vi "synchronize with binary serial stream.vi"() -> ()   [LabVIEW 2017]
uses:
  typedefs/reading.ctl
  typedefs/readingType.ctl
  typedefs/bytes in a reading.ctl
panel:
  out "first reading":T1
  in  "error in":errorcluster
  in  "serial port":refnum<visa-resource-name>
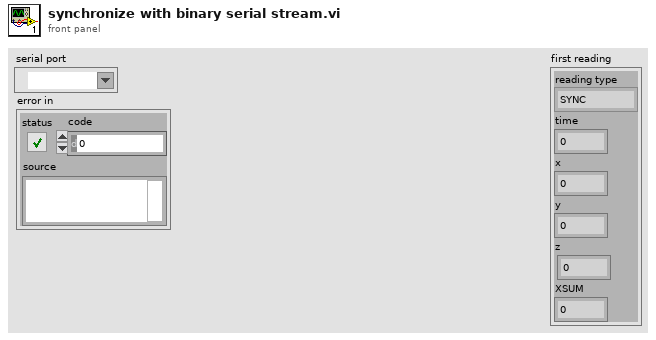
[diagram p1: front panel]
types:
  T1 = typedef "reading.ctl" = cluster{"reading type":T2, "time":fxp<+,48,48>, "x":sgl, "y":sgl, "z":sgl, "XSUM":u8}
  T2 = typedef "readingType.ctl" = enum8{"SYNC", "DETVAL", "COILI", "MAGVEC", "ACCVEC"}
  T3 = enum16{"big-endian, network order", "native, host order", "little-endian"}
  T4 = typedef "bytes in a reading.ctl" = u32
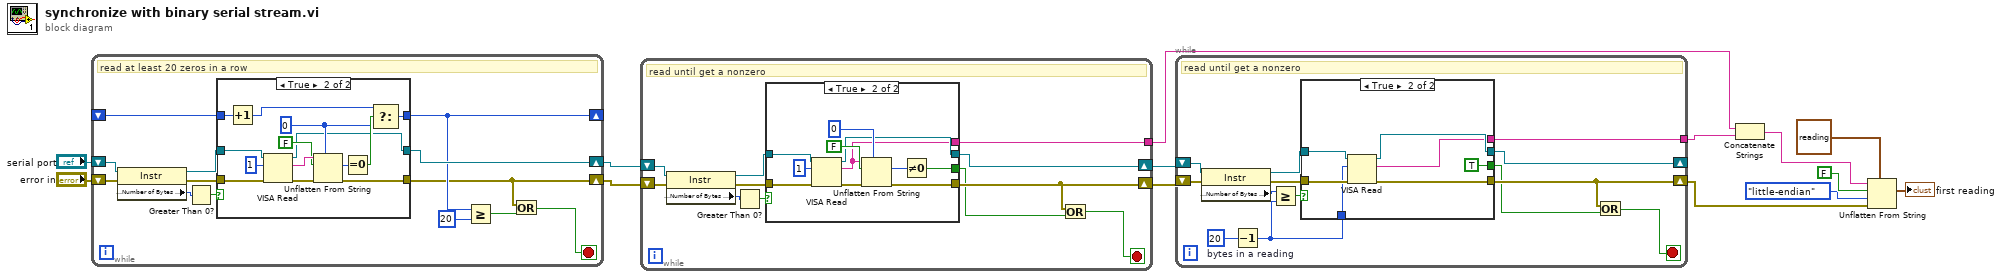
[diagram p0: block diagram]
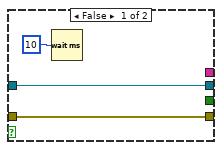
[diagram p2: hidden frame]
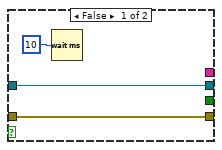
[diagram p3: hidden frame]
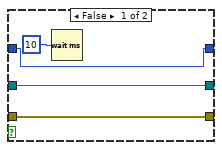
[diagram p4: hidden frame]
diagram:
  n1 = while {
    shift-right: [w19] -> _
    shift-left: _ -> [w22]
    shift-right: [w21] -> w11
    shift-left: "serial port" -> [w27]
    shift-right: [w16] -> w12
    shift-left: "error in" -> [w20]
    stop <- w15 stop-if-true
    # "read at least 20 zeros in a row"
    n2 = property class="Instr"(reference=w27, error in=w20) -> (reference out=w24:refnum<visa-resource-name>, error out=w23:errorcluster, "Serial Settings:Number of Bytes at Serial Port"=w26:u32)
    n3 = Greater Than 0?(x=w26) -> (x > 0?=w25:bool)
    n4 = case shown="True" w25 {
      tunnel: w24 -> [w28 w45]
      tunnel: w23 -> [w29 w43]
      tunnel: [w30 w36] -> w19
      tunnel: w22 -> [w30 w34]
      tunnel: [w28 w33] -> w21
      tunnel: [w29 w32] -> w16
      frame False {
        n5 = Wait (ms)(milliseconds to wait=u32 10) -> ()  [unwired: 1 out]
      }
      frame True {
        w37 = u8 0
        n6 = Increment(x=w34) -> (x+1=w35:u8)
        n7 = VISA Read(VISA resource name=w45, byte count=u32 1, error in (no error)=w43) -> (VISA resource name out=w33:refnum<visa-resource-name>, read buffer=w42:string, error out=w40:errorcluster)  [unwired: 1 out]
        n8 = Unflatten From String(type=w37, binary string=w42, data includes array or string size? (T)=FALSE, error in (no error)=w40) -> (value=w39:u8, error out=w32:errorcluster)  [unwired: 1 in, 1 out]
        n9 = Equal To 0?(x=w39) -> (x = 0?=w38:bool)
        n10 = Select(t=w35, s=w38, f=w37) -> (s? t:f=w36:u8)
      }
    }
    n11 = Greater Or Equal?(x=w19, y=u8 20) -> (x >= y?=w17:bool)
    n12 = Or(x=w16, y=w17) -> (x .or. y?=w15:bool)
  }
  n13 = while {
    shift-right: [w51] -> w9
    shift-left: w11 -> [w56]
    shift-right: [w49] -> w10
    shift-left: w12 -> [w50]
    tunnel: [w47] -> w7
    stop <- w48 stop-if-true
    # "read until get a nonzero"
    n14 = property class="Instr"(reference=w56, error in=w50) -> (reference out=w53:refnum<visa-resource-name>, error out=w52:errorcluster, "Serial Settings:Number of Bytes at Serial Port"=w55:u32)
    n15 = Greater Than 0?(x=w55) -> (x > 0?=w54:bool)
    n16 = case shown="True" w54 {
      tunnel: w53 -> [w57 w70]
      tunnel: w52 -> [w58 w68]
      tunnel: [w57 w64] -> w51
      tunnel: [w58 w63] -> w49
      tunnel: [_ w62] -> w47
      tunnel: [_ w60] -> w46
      frame False {
        n17 = Wait (ms)(milliseconds to wait=u32 10) -> ()  [unwired: 1 out]
      }
      frame True {
        n18 = VISA Read(VISA resource name=w70, byte count=u32 1, error in (no error)=w68) -> (VISA resource name out=w64:refnum<visa-resource-name>, read buffer=w62:string, error out=w66:errorcluster)  [unwired: 1 out]
        n19 = Unflatten From String(type=u8 0, binary string=w62, data includes array or string size? (T)=FALSE, error in (no error)=w66) -> (value=w61:u8, error out=w63:errorcluster)  [unwired: 1 in, 1 out]
        n20 = Not Equal To 0?(x=w61) -> (x != 0?=w60:bool)
      }
    }
    n21 = Or(x=w49, y=w46) -> (x .or. y?=w48:bool)
  }
  n22 = while {
    shift-right: [w79] -> _
    shift-left: w9 -> [w83]
    shift-right: [w77] -> w2
    shift-left: w10 -> [w78]
    tunnel: [w75] -> w8
    stop <- w76 stop-if-true
    w73 = T4 20  # bytes in a reading
    # "read until get a nonzero"
    n23 = property class="Instr"(reference=w83, error in=w78) -> (reference out=w81:refnum<visa-resource-name>, error out=w80:errorcluster, "Serial Settings:Number of Bytes at Serial Port"=w72:u32)
    n24 = Decrement(x=w73) -> (x-1=w71:T4)
    n25 = Greater Or Equal?(x=w72, y=w71) -> (x >= y?=w82:bool)
    n26 = case shown="True" w82 {
      tunnel: w81 -> [w84 w93]
      tunnel: w80 -> [w85 w92]
      tunnel: [w84 w91] -> w79
      tunnel: [w85 w90] -> w77
      tunnel: [_ w89] -> w75
      tunnel: [_ TRUE] -> w74
      tunnel: w71 -> [_ w87]
      frame False {
        n27 = Wait (ms)(milliseconds to wait=u32 10) -> ()  [unwired: 1 out]
      }
      frame True {
        n28 = VISA Read(VISA resource name=w93, byte count=w87, error in (no error)=w92) -> (VISA resource name out=w91:refnum<visa-resource-name>, read buffer=w89:string, error out=w90:errorcluster)  [unwired: 1 out]
      }
    }
    n29 = Or(x=w77, y=w74) -> (x .or. y?=w76:bool)
  }
  n30 = Concatenate Strings(w7, w8) -> (w6:string)
  n31 = Unflatten From String(type=T1 {"reading type"=enum."SYNC", "time"=0.0, "x"=0.0, "y"=0.0, "z"=0.0, "XSUM"=0} ("reading"), binary string=w6, data includes array or string size? (T)=FALSE, byte order (0:big-endian, network order)=T3."little-endian", error in (no error)=w2) -> (value=→"first reading":T1)  [unwired: 2 out]
